vi "Tempersture Warning.vi"() -> ()   [LabVIEW 2014]
panel:
  out "Warning Text":string
  in  "Min temp":dbl
  in  "Max Temp":dbl
  in  "Current Temp":dbl
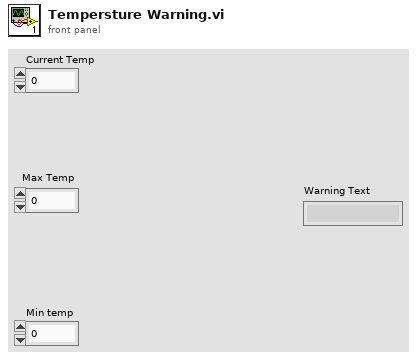
[diagram p1: front panel]
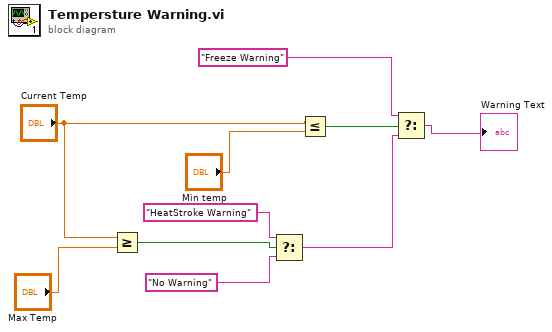
[diagram p0: block diagram]
diagram:
  n1 = Greater Or Equal?(x="Current Temp", y="Max Temp") -> (x >= y?=w6:bool)
  n2 = Select(t="HeatStroke Warning", s=w6, f="No Warning") -> (s? t:f=w5:string)
  n3 = Less Or Equal?(x="Current Temp", y="Min temp") -> (x <= y?=w7:bool)
  n4 = Select(t="Freeze Warning", s=w7, f=w5) -> (s? t:f=→"Warning Text":string)
